vi "Merge Directories__ogtk_withSubDirFilter.vi"(4 "Subdir filter (\"\": none)":string, 6 "Ignore Read-Only? (FALSE)":bool, 7 "Delete Source? (FALSE)":bool, 8 "error in (no error)":errorcluster, 9 "Overwrite Existing Files? (FALSE)":bool, 10 "target directory path":path, 11 "source directory path":path) -> (0 "error out":errorcluster, 3 "dup target directory path":path)   [LabVIEW 2010]
doc: "Copies the contents of source directory into the destination directory. If source directory has subdirectories they will be copied into the destination directory recursively. Optionally, existing files may be overwritten, by setting the \"Overwrite Existing Files?\" input to TRUE. If you attempt to overwrite an existing file without setting to TRUE ans error will be returned. If FALSE, existing files will not be overwritten and no error wil be returned, Optionally, read-only files may be overwritten, by setting the \"Ignore Read-Only?\" input to TRUE. If you attempt to overwrite a read-only files without setting to TRUE an error will be returned. Optionally, by setting the \"Delete Source?\" input to TRUE the source directory will be deleted upon merge completion if no errors occured."
uses:
  <userlib>/_OpenG.lib/file/file.llb/Build Path - File Names Array__ogtk.vi
  <userlib>/_OpenG.lib/array/array.llb/Filter 1D Array with Scalar (String)__ogtk.vi
  <userlib>/_OpenG.lib/file/file.llb/Compare Two Paths - Scalar__ogtk.vi
  <userlib>/_OpenG.lib/file/file.llb/Build Path - Traditional - path__ogtk.vi
  <userlib>/_OpenG.lib/file/file.llb/Strip Path - Traditional__ogtk.vi
panel:
  # "OpenG Library.vi\n\nMerge Directories.vi\n\nCopies the contents of source directory into the destination directory.\n\nPlease visit http://www.OpenG.org to learn about the\nOpen Source LabVIEW software movement.\n\nNOTICE -- YOU MUST LEAVE THIS NOTICE IN PLACE.  PER THE TERMS OF THE LICENSE BELOW, YOU MAY SUBLICENSE THIS SOFTWARE \nIN ANY WAY THAT DOES NOT CONFLICT WITH THIS LICENSE.\n\n### BSD License (http://www.opensource.org/licenses/bsd-license.php) Begin ###\n \nCopyright (c) 2002-2004, Jim Kring <jim@jimkring.com>\nCopyright (c) 2002, Cal-Bay Systems, Inc. <info@calbay.com>\n\nAll rights reserved.\n\nRedistribution and use in source and binary forms, with or without modification, are permitted provided that the following conditions are met:\n\n    * Redistributions of source code must retain the above copyright notice, this list of conditions and the following disclaimer.\n    * Redistributions in binary form must reproduce the above copyright notice, this list of conditions and the following disclaimer in the \n       documentation and/or other materials provided with the distribution.\n    * Neither the name of SciWare, James Kring, Inc., nor the names of its contributors may be used to endorse or promote products derived \n       from this software without specific prior written permission.\n\nTHIS SOFTWARE IS PROVIDED BY THE COPYRIGHT HOLDERS AND CONTRIBUTORS \"AS IS\" AND ANY EXPRESS OR IMPLIED WARRANTIES, \nINCLUDING, BUT NOT LIMITED TO, THE IMPLIED WARRANTIES OF MERCHANTABILITY AND FITNESS FOR A PARTICULAR PURPOSE ARE \nDISCLAIMED. IN NO EVENT SHALL THE COPYRIGHT OWNER OR CONTRIBUTORS BE LIABLE FOR ANY DIRECT, INDIRECT, INCIDENTAL,\n SPECIAL, EXEMPLARY, OR CONSEQUENTIAL DAMAGES (INCLUDING, BUT NOT LIMITED TO, PROCUREMENT OF SUBSTITUTE GOODS OR \nSERVICES; LOSS OF USE, DATA, OR PROFITS; OR BUSINESS INTERRUPTION) HOWEVER CAUSED AND ON ANY THEORY OF LIABILITY, \nWHETHER IN CONTRACT, STRICT LIABILITY, OR TORT (INCLUDING NEGLIGENCE OR OTHERWISE) ARISING IN ANY WAY OUT OF THE USE \nOF THIS SOFTWARE, EVEN IF ADVISED OF THE POSSIBILITY OF SUCH DAMAGE.\n\n### BSD License End ###"
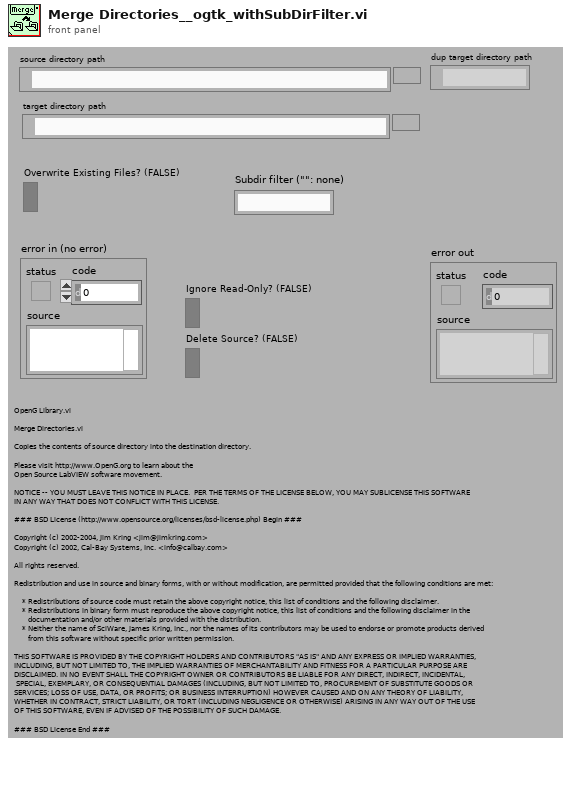
[diagram p1: front panel]
types:
  T1 = cluster{"Archive":bool, "Normal":bool, "Temporary":bool, "Compressed":bool, "Offline":bool, "Content Indexed":bool, "Encrypted (cannot set)":bool}
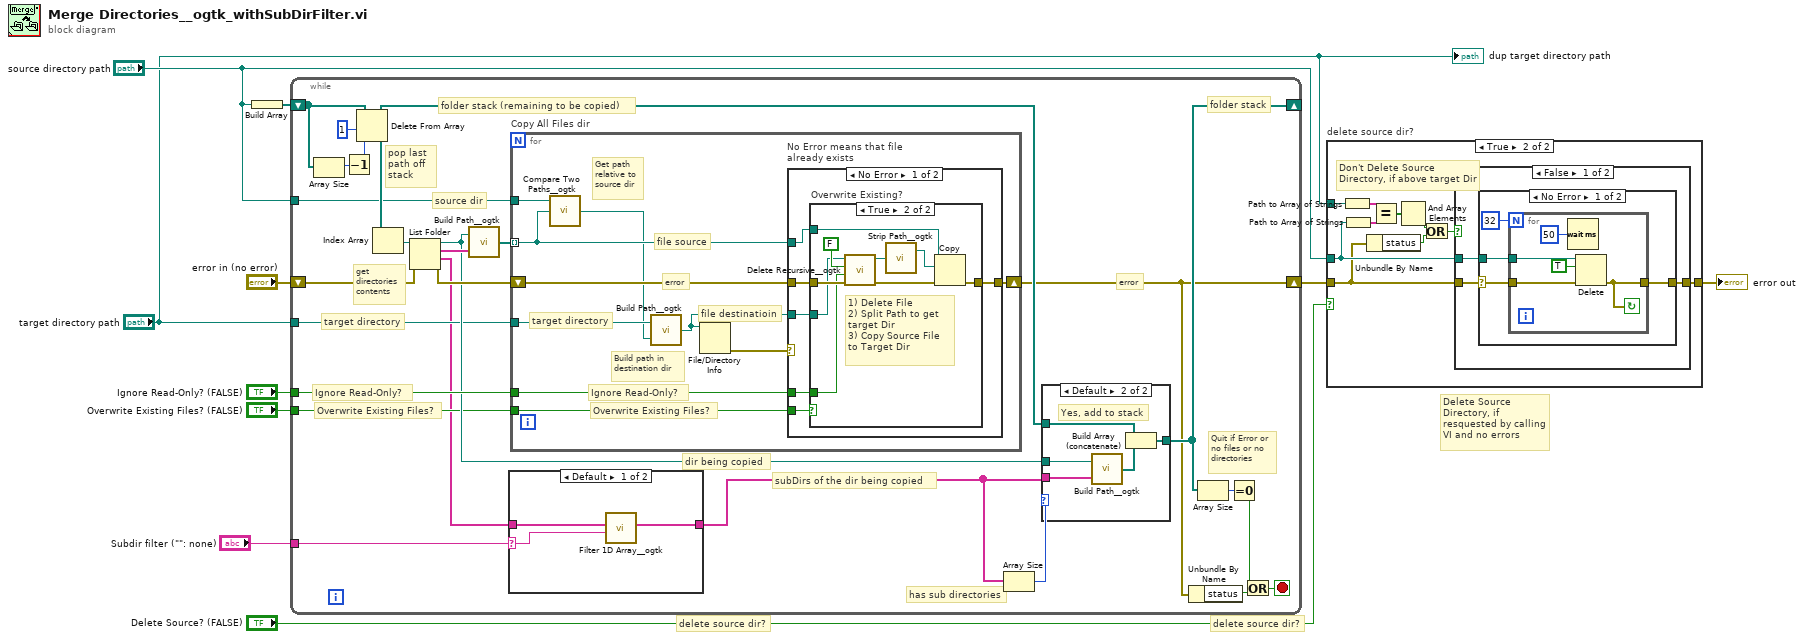
[diagram p0: block diagram]
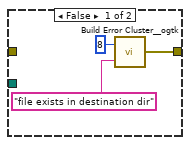
[diagram p4: hidden frame]
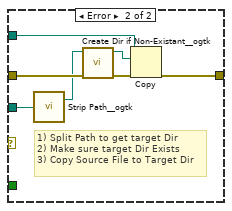
[diagram p5: hidden frame]
diagram:
  # "Delete Source Directory, if resquested by calling VI and no errors"
  # "delete source dir?"
  # "delete source dir?"
  n1 = Build Array("source directory path") -> (w9:path[])
  n2 = while {
    shift-right: [w22] -> _
    shift-left: w9 -> [w25]
    shift-right: [w14] -> w6
    shift-left: "error in (no error)" -> [w26]
    tunnel: "Ignore Read-Only? (FALSE)" -> [w21]
    tunnel: "source directory path" -> [w17]
    tunnel: "target directory path" -> [w16]
    tunnel: "Overwrite Existing Files? (FALSE)" -> [w15]
    tunnel: "Subdir filter (\"\": none)" -> [w13]
    stop <- w27 stop-if-true
    (unwired) T1 {"Archive"=FALSE, "Normal"=FALSE, "Temporary"=FALSE, "Compressed"=FALSE, "Offline"=FALSE, "Content Indexed"=FALSE, "Encrypted (cannot set)"=FALSE} ("FileAttribute")
    # "folder stack"
    # "error"
    # "Overwrite Existing Files?"
    # "Ignore Read-Only?"
    # "target directory"
    # "subDirs of the dir being copied"
    # "dir being copied"
    # "folder stack (remaining to be copied)"
    # "source dir"
    # "get directories contents"
    # "pop last path off stack"
    # "Quit if Error or no files or no directories"
    # "has sub directories"
    n3 = Array Size(array=w25) -> (size(s)=w23:i32)
    n4 = Decrement(x=w23) -> (x-1=w24:i32)
    n5 = Delete From Array(array=w25, length=1 ("Length"), index=w24) -> (deleted portion=w35:path[], array with subset deleted=w31:path[])
    n6 = Index Array(array=w35) -> (element=w34:path)  [unwired: 1 in]
    n7 = List Folder(path=w34, error in=w26) -> (path out=w19:path, filenames=w20:string[], folder names=w12:string[], error out=w33:errorcluster)  [unwired: 2 in]
    n8 = call-poly <userlib>:"Build Path__ogtk.vi"("name or relative path"=w20, "base path"=w19) -> ("appended path"=w18:path[])
    n9 = case shown="Default" w13 {
      selector: w13 -> [w38 _]
      tunnel: w12 -> [w39 w40]
      tunnel: [w37 w40] -> w11
      frame Default {
        n10 = call-poly <userlib>:"Filter 1D Array__ogtk.vi"("items to filter"=w38, "array"=w39) -> ("filtered array"=w37:string[])  [unwired: 4 in, 1 out]
      }
      frame "" {
      }
    }
    n11 = for "Copy All Files dir" {
      shift-right: [w52] -> w14
      shift-left: w33 -> [w53]
      tunnel: w21 -> [w50]
      tunnel: w18 -> [w48] mode=indexing
      tunnel: w17 -> [w49]
      tunnel: w16 -> [w56]
      tunnel: w15 -> [w51]
      # "Ignore Read-Only?"
      # "Overwrite Existing Files?"
      # "file destinatioin"
      # "file source"
      # "target directory"
      # "error"
      # "Build path in destination dir"
      # "Get path relative to source dir"
      n12 = call-poly <userlib>:"Compare Two Paths__ogtk.vi"("path2"=w48, "path1"=w49) -> ("relative path from 1 to 2"=w47:path)  [unwired: 1 in, 2 out]
      n13 = call-poly <userlib>:"Build Path__ogtk.vi"("name or relative path"=w47, "base path"=w56) -> ("appended path"=w54:path)
      n14 = File/Directory Info(path=w54) -> (error out=w55:errorcluster)  [unwired: 1 in, 6 out]
      n15 = case "No Error means that file\nalready exists" shown="No Error" w55 {
        tunnel: w54 -> [w59 w79]
        tunnel: w48 -> [w58 w81]
        tunnel: w53 -> [w61 w78]
        tunnel: [w60 w80] -> w52
        tunnel: w51 -> [w62 _]
        tunnel: w50 -> [w57 _]
        frame No Error {
          n16 = case "Overwrite Existing?" shown="True" w62 {
            tunnel: w61 -> [_ w74]
            tunnel: [w63 w72] -> w60
            tunnel: w59 -> [_ w68]
            tunnel: w58 -> [_ w71]
            tunnel: w57 -> [_ w70]
            frame False {
              n17 = call <userlib>:"Build Error Cluster__ogtk.vi"("String to Prepend to source (\"\")"="file exists in destination dir" ("String to Prepend to source (\"\")"), "code"=8) -> ("error out"=w63:errorcluster)
            }
            frame True {
              # "1) Delete File\n2) Split Path to get target Dir\n3) Copy Source File to Target Dir"
              n18 = call <userlib>:"Delete Recursive__ogtk.vi"("error in (no error)"=w74, "Ignore Read-Only? (FALSE)"=w70, "Recursive? (FALSE)"=FALSE, "Path"=w68) -> ("error out"=w73:errorcluster, "dup Path"=w67:path)  [unwired: 6 in]
              n19 = call-poly <userlib>:"Strip Path__ogtk.vi"("path"=w67) -> ("stripped path"=w66:path)  [unwired: 1 out]
              n20 = Copy(8:w73, 10:w66, 11:w71) -> (0:w72:errorcluster)  [unwired: 2 in, 2 out]
            }
          }
        }
        frame Error {
          # "1) Split Path to get target Dir\n2) Make sure target Dir Exists\n3) Copy Source File to Target Dir"
          n21 = call-poly <userlib>:"Strip Path__ogtk.vi"("path"=w79) -> ("stripped path"=w75:path)  [unwired: 1 out]
          n22 = call <userlib>:"Create Dir if Non-Existant__ogtk.vi"("error in (no error)"=w78, "Directory Path"=w75) -> ("error out"=w77:errorcluster, "dup Directory Path"=w76:path)  [unwired: 7 in, 1 out]
          n23 = Copy(8:w77, 10:w76, 11:w81) -> (0:w80:errorcluster)  [unwired: 2 in, 2 out]
        }
      }
    }
    n24 = Array Size(array=w11) -> (size(s)=w32:i32)
    n25 = case shown="Default" w32 {
      tunnel: w19 -> [_ w42]
      tunnel: w11 -> [_ w46]
      tunnel: w31 -> [w41 w44]
      tunnel: [w41 w43] -> w22
      frame 0 {
      }
      frame Default {
        # "Yes, add to stack"
        n26 = call-poly <userlib>:"Build Path__ogtk.vi"("name or relative path"=w46, "base path"=w42) -> ("appended path"=w45:path[])
        n27 = Build Array (concatenate)(w44, w45) -> (w43:path[])
      }
    }
    n28 = Unbundle By Name(w14) -> ("status"=w29:bool)
    n29 = Array Size(array=w22) -> (size(s)=w30:i32)
    n30 = Equal To 0?(x=w30) -> (x = 0?=w28:bool)
    n31 = Or(x=w28, y=w29) -> (x .or. y?=w27:bool)
  }
  n32 = case "delete source dir?" shown="True" "Delete Source? (FALSE)" {
    tunnel: w6 -> [w82 w86]
    tunnel: [w82 w92] -> w5
    tunnel: "source directory path" -> [_ w90]
    tunnel: "target directory path" -> [_ w91]
    frame False {
    }
    frame True {
      # "Don't Delete Source Directory, if above target Dir"
      n33 = Path to Array of Strings(0:w91) -> (2:w89:string[])  [unwired: 1 out]
      n34 = Path to Array of Strings(0:w90) -> (2:w88:string[])  [unwired: 1 out]
      n35 = Unbundle By Name(w86) -> ("status"=w83:bool)
      n36 = Equal?(x=w89, y=w88) -> (x = y?=w87:bool[])
      n37 = And Array Elements(Boolean array=w87) -> (logical AND=w85:bool)
      n38 = Or(x=w85, y=w83) -> (x .or. y?=w84:bool)
      n39 = case shown="False" w84 {
        tunnel: w90 -> [w95 _]
        tunnel: [w94 w106] -> w92
        tunnel: w86 -> [w93 w106]
        frame False {
          n40 = case shown="No Error" w93 {
            selector: w93 -> [w97 w105]
            tunnel: w95 -> [w99 _]
            tunnel: [w98 w105] -> w94
            frame No Error {
              n41 = for {
                N: 32 -> [_]
                tunnel: w99 -> [w104]
                tunnel: [w100] -> w98
                tunnel: w97 -> [w102]
                stop <- w100 continue-if-true
                n42 = Wait (ms)(milliseconds to wait=u32 50) -> ()  [unwired: 1 out]
                n43 = Delete(path (use dialog)=w104, entire hierarchy (F)=TRUE, error in=w102) -> (error out=w100:errorcluster)  [unwired: 2 in, 2 out]
              }
            }
            frame Error {
            }
          }
        }
        frame True {
        }
      }
    }
  }
  "error out" <- w5
  "dup target directory path" <- "target directory path"
